vi "Update Value.vi"(6 "Time":dbl, 8 "error in (no error)":errorcluster, 11 "NumericIndicator in":refnum<class "NumericIndicator.lvclass">) -> (0 "error out":errorcluster, 1 "Update":bool, 2 "Value":variant, 3 "NumericIndicator out":refnum<class "NumericIndicator.lvclass">)   [LabVIEW 2020, in "VolatusGUIElements.lvlib" / "NumericIndicator.lvclass"]
uses:
  NumericIndicator.lvclass
  NumericIndicator.lvclass/NumericIndicator.ctl
  lv-vecto/Vecto/Channel/Channel.lvclass/Channel.ctl
  lv-vecto/Vecto/Group/Value by Index.vi
  lv-vecto/Vecto/Channel/Channel.lvclass
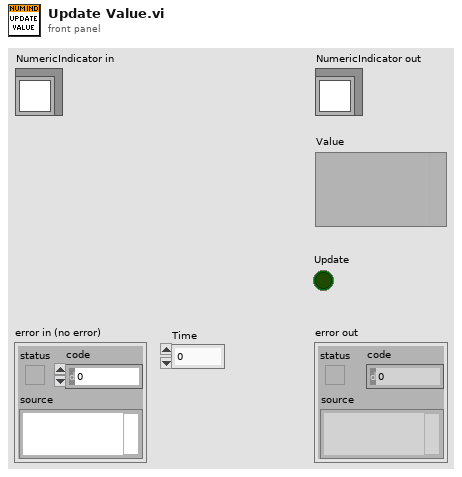
[diagram p1: front panel]
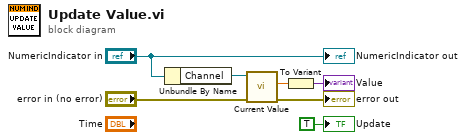
[diagram p0: block diagram]
diagram:
  n1 = Unbundle By Name("NumericIndicator in") -> ("Channel"=w5:refnum<class "Channel.lvclass">)
  n2 = call "Current Value.vi"("error in (no error)"="error in (no error)", "Channel in"=w5) -> ("error out"=→"error out":errorcluster, "Scaled"=w4:dbl)  [unwired: 5 in, 3 out]
  n3 = To Variant(anything=w4) -> (Variant=→"Value":variant)
  "NumericIndicator out" <- "NumericIndicator in"
  "Update" <- TRUE ("Update")
